vi "Get config path.vi"(8 "error in":errorcluster) -> (0 "error out":errorcluster, 1 "Cassette codes":i32[](array[numeric]), 2 "Family names":string[](array[string]), 3 "Variants":string[](array[string]))   [LabVIEW 2023]
uses:
  <vilib>/Utility/config.llb/Read Key (I32).vi
  <vilib>/Utility/config.llb/Read Key (String).vi
  <vilib>/Utility/config.llb/NI_LVConfig.lvlib
panel:
  out "key names":string[](array[string])
  out "appended path":path
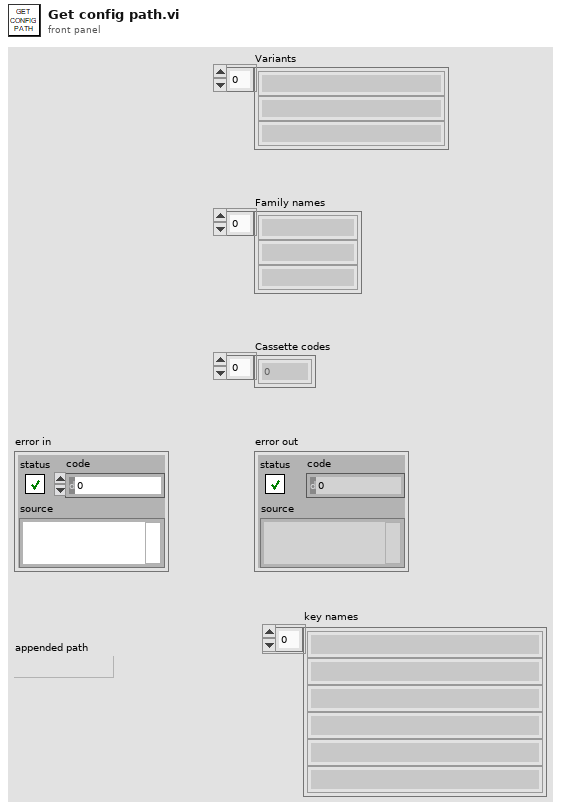
[diagram p1: front panel]
types:
  T1 = typedef "NI_LVConfig.lvlib/Config Data RefNum.ctl" = refnum<k1>
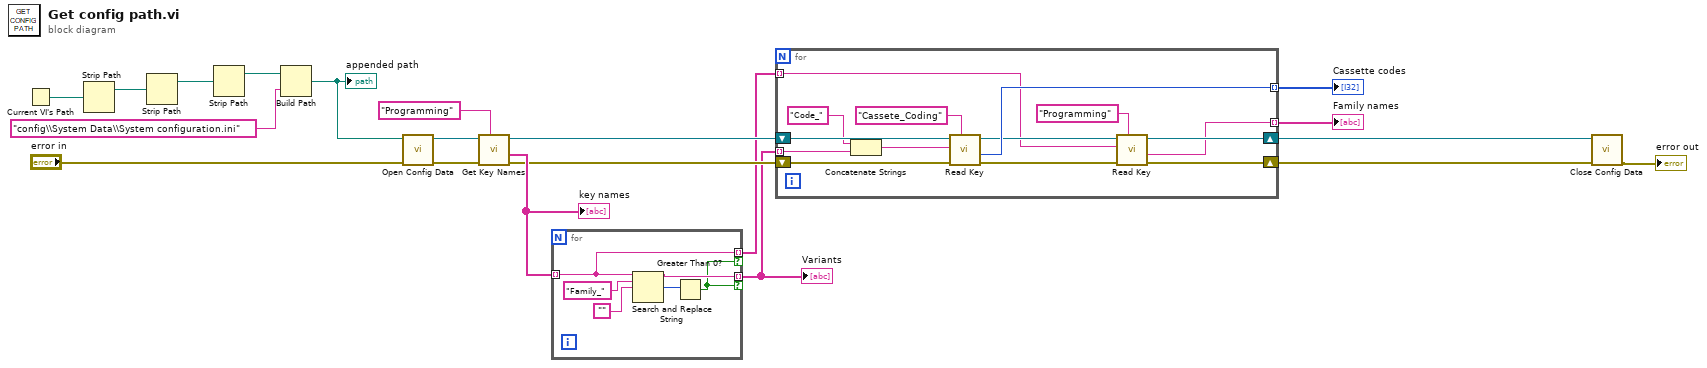
[diagram p0: block diagram]
diagram:
  n1 = Current VI's Path() -> (path=w16:path)
  n2 = Strip Path(path=w16) -> (stripped path=w17:path)  [unwired: 1 out]
  n3 = Strip Path(path=w17) -> (stripped path=w18:path)  [unwired: 1 out]
  n4 = Strip Path(path=w18) -> (stripped path=w19:path)  [unwired: 1 out]
  n5 = Build Path(base path=w19, name or relative path="config\\System Data\\System configuration.ini") -> (appended path=w15:path)
  "appended path" <- w15
  n6 = call <vilib>:"Open Config Data.vi"("error in (no error)"="error in", "configuration file path"=w15) -> ("error out"=w13:errorcluster, "refnum"=w14:T1)  [unwired: 7 in, 1 out]
  n7 = call <vilib>:"Get Key Names.vi"("section"="Programming", "error in (no error)"=w13, "refnum"=w14) -> ("error out"=w7:errorcluster, "key names"=w11:string[], "refnum out"=w8:T1)  [unwired: 5 in, 1 out]
  "key names" <- w11
  n8 = for {
    tunnel: w11 -> [w22] mode=indexing
    tunnel: [w23] -> w4 mode=indexing if=w21
    tunnel: [w22] -> w2 mode=indexing if=w21
    n9 = Search and Replace String(input string=w22, search string="Family_", replace string="") -> (result string=w23:string, number of replacements=w24:i32)  [unwired: 5 in, 2 out]
    n10 = Greater Than 0?(x=w24) -> (x > 0?=w21:bool)
  }
  "Variants" <- w4
  n11 = for {
    shift-right: [w32] -> w5
    shift-left: w8 -> [w40]
    shift-right: [w30] -> w6
    shift-left: w7 -> [w39]
    tunnel: w4 -> [w37] mode=indexing
    tunnel: [w34] -> w3 mode=indexing
    tunnel: w2 -> [w29] mode=indexing
    tunnel: [w27] -> w1 mode=indexing
    n12 = Concatenate Strings("Code_" ("string"), w37) -> (w36:string)
    n13 = call-poly <vilib>:"Read Key.vi"("section"="Cassete_Coding", "error in (no error)"=w39, "key"=w36, "refnum"=w40) -> ("error out"=w31:errorcluster, "value"=w34:i32, "refnum out"=w33:T1)  [unwired: 4 in, 1 out]
    n14 = call-poly <vilib>:"Read Key.vi"("section"="Programming", "error in (no error)"=w31, "key"=w29, "refnum"=w33) -> ("error out"=w30:errorcluster, "value"=w27:string, "refnum out"=w32:T1)  [unwired: 4 in, 1 out]
  }
  "Family names" <- w1
  "Cassette codes" <- w3
  n15 = call <vilib>:"Close Config Data.vi"("error in (no error)"=w6, "refnum"=w5) -> ("error out"=→"error out":errorcluster)  [unwired: 8 in, 1 out]
